vi "CursorDriver.vi"   [LabVIEW 2014]
uses:
  User32.dll
panel:
  # "Wiggle Driver"
types:
  T1 = typedef "LVRectTypeDef.ctl" = cluster{"Left":i16, "Top":i16, "Right":i16, "Bottom":i16}
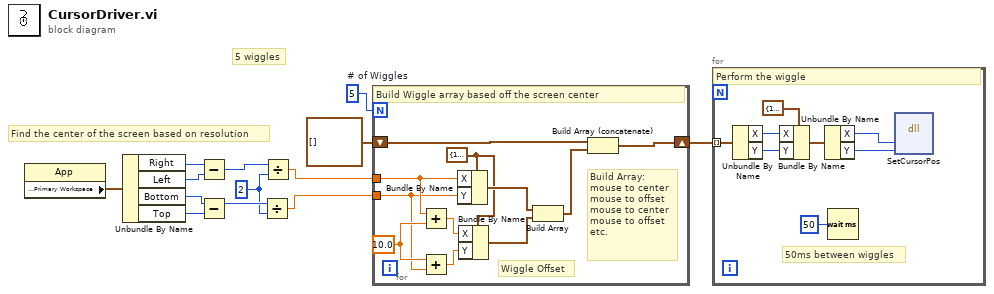
[diagram p0: block diagram]
diagram:
  w5 = 5  # # of Wiggles
  w6 = i16 2 ("y")
  # "5 wiggles"
  # "Find the center of the screen based on resolution"
  n1 = property class="App"() -> ("Display:Primary Workspace"=w13:T1)  [unwired: 2 in, 2 out]
  n2 = Unbundle By Name(w13) -> ("Right"=w12:i16, "Left"=w11:i16, "Bottom"=w10:i16, "Top"=w9:i16)
  n3 = Subtract(x=w12, y=w11) -> (x-y=w8:i16)
  n4 = Subtract(x=w10, y=w9) -> (x-y=w7:i16)
  n5 = Divide(x=w7, y=w6) -> (x/y=w3:dbl)
  n6 = Divide(x=w8, y=w6) -> (x/y=w4:dbl)
  n7 = for {
    N: w5 -> [_]
    tunnel: w4 -> [w17]
    tunnel: w3 -> [w16]
    shift-right: [w19] -> w1
    shift-left: cluster{"X":i32, "Y":i32}[] [] -> [w22]
    w18 = 10.0 ("y")
    w23 = cluster{"X":i32, "Y":i32} {"X"=1001, "Y"=1000} ("Cluster")
    # "Build Array:\nmouse to center\nmouse to offset\nmouse to center\nmouse to offset\netc."
    # "Wiggle Offset"
    # "Build Wiggle array based off the screen center"
    n8 = Add(x=w17, y=w18) -> (x+y=w15:dbl)
    n9 = Add(x=w18, y=w16) -> (x+y=w14:dbl)
    n10 = Bundle By Name(cluster=w23, "X"=w17, "Y"=w16) -> (w24:cluster{"X":i32, "Y":i32})
    n11 = Bundle By Name(cluster=w23, "X"=w15, "Y"=w14) -> (w21:cluster{"X":i32, "Y":i32})
    n12 = Build Array(w24, w21) -> (w20:cluster{"X":i32, "Y":i32}[])
    n13 = Build Array (concatenate)(w22, w20) -> (w19:cluster{"X":i32, "Y":i32}[])
  }
  n14 = for {
    tunnel: w1 -> [w28] mode=indexing
    # "50ms between wiggles"
    # "Perform the wiggle"
    n15 = Unbundle By Name(w28) -> ("X"=w27:i32, "Y"=w26:i32)
    n16 = Bundle By Name(cluster=cluster{"X":i32, "Y":i32} {"X"=1001, "Y"=1000} ("Cluster"), "X"=w27, "Y"=w26) -> (w32:cluster{"X":i32, "Y":i32})
    n17 = Unbundle By Name(w32) -> ("X"=w29:i32, "Y"=w30:i32)
    n18 = Wait (ms)(milliseconds to wait=u32 50) -> ()  [unwired: 1 out]
    n19 = dll-call lib="user32.dll" fn="SetCursorPos"("dx"=w29, "dy"=w30) -> ()  [unwired: 6 in, 2 out]
  }
